vi "Get Identifier.vi"(8 "error in (no error)":errorcluster, 11 "Execution Unit Implementation in":refnum<class "Execution Unit Implementation.lvclass">) -> (0 "error out":errorcluster, 2 "Identifier":string, 3 "Execution Unit Implementation out":refnum<class "Execution Unit Implementation.lvclass">)   [LabVIEW 2020, in "Communication Bus Template Engine.lvlib" / "Implementation.lvlib" / "Execution Unit Implementation.lvclass"]
uses:
  Execution Unit Implementation.lvclass
  Execution Unit Implementation.lvclass/Execution Unit Implementation.ctl
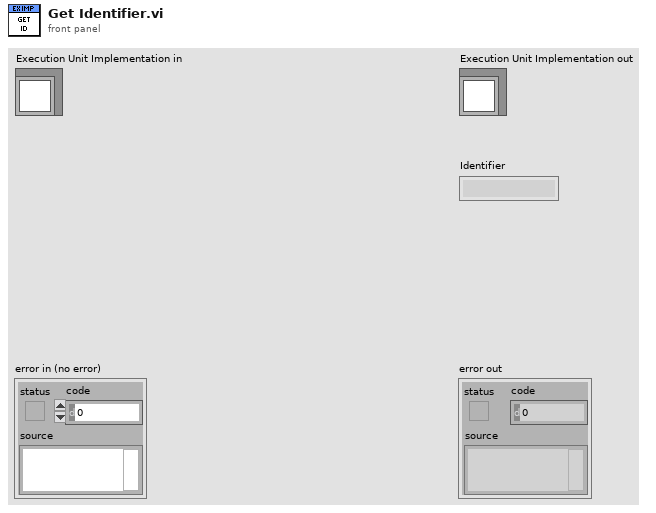
[diagram p1: front panel]
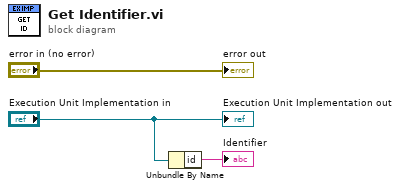
[diagram p0: block diagram]
diagram:
  n1 = Unbundle By Name("Execution Unit Implementation in") -> ("id"=→"Identifier":string)
  "error out" <- "error in (no error)"
  "Execution Unit Implementation out" <- "Execution Unit Implementation in"
